vi "channeldata_2ch.vi"() -> ()   [LabVIEW 2019]
panel:
  out "Error Out":errorcluster
  in  "TDMS File":path=path "C:/Python/projects/nitdms/tests/tdms_files/channeldata_2ch.tdms"
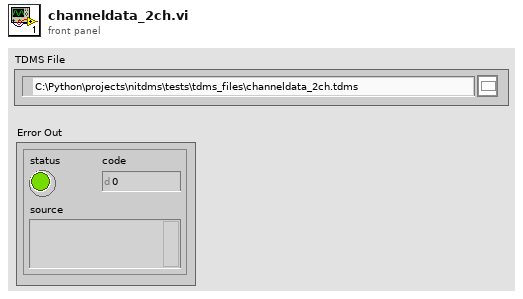
[diagram p1: front panel]
types:
  T1 = enum16{"open", "open or create", "create or replace", "create", "open (read-only)"}
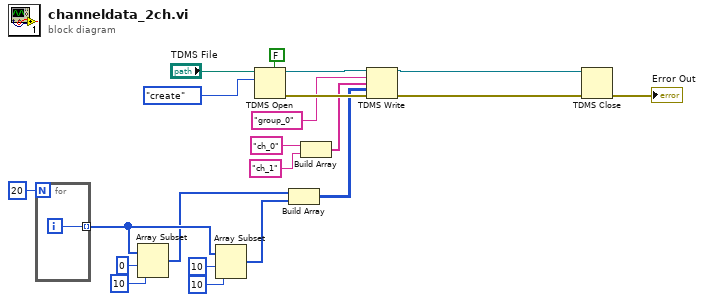
[diagram p0: block diagram]
diagram:
  n1 = for {
    N: 20 -> [_]
    tunnel: [w22] -> w9 mode=indexing
    i -> [w22]
  }
  n2 = Array Subset(array=w9, index=0, length=10) -> (w8:i32[])
  n3 = Array Subset(array=w9, index=10, length=10) -> (w7:i32[])
  n4 = TDMS Open(5:FALSE ("create index file? (T)"), 10:T1."create" ("operation (0:open)"), 11:"TDMS File") -> (0:w17:errorcluster, 3:w16:refnum<k34>)  [unwired: 4 in]
  n5 = Build Array(w8, w7) -> (w3:i32[][])
  n6 = Build Array("ch_0", "ch_1") -> (w4:string[])
  n7 = TDMS Write(0:w16, 5:"group_0", 7:w4, 9:w3, 11:w17) -> (4:w1:refnum<k34>, 15:w2:errorcluster)  [unwired: 1 in, 2 out]
  n8 = TDMS Close(8:w2, 11:w1) -> (0:→"Error Out":errorcluster)  [unwired: 1 out]
